vi "Resize Xcontrol.vi"(8 "error in (no error)":errorcluster, 10 "Big size":bool, 11 "reference":refnum<vi>) -> (0 "error out":errorcluster)   [LabVIEW 2015]
uses:
  <vilib>/Utility/miscctls.llb/LVBoundsTypeDef.ctl
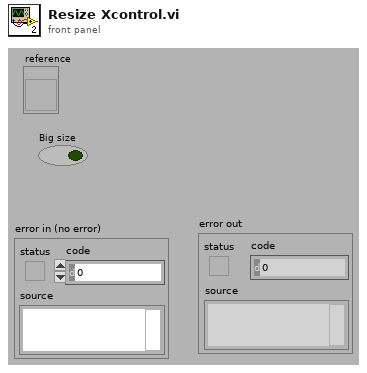
[diagram p1: front panel]
types:
  T1 = typedef "LVBoundsTypeDef.ctl" = cluster{"Width":u32, "Height":u32}
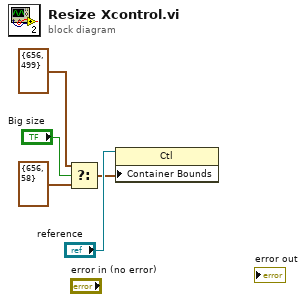
[diagram p0: block diagram]
diagram:
  n1 = Select(t=T1 {"Width"=656, "Height"=499} ("XControl:Container Bounds"), s="Big size", f=T1 {"Width"=656, "Height"=58} ("XControl:Container Bounds")) -> (s? t:f=w1:T1)
  n2 = property class="Ctl"(reference="reference", "Container Bounds"=w1) -> ()  [unwired: 1 in, 2 out]
